vi "Begin.vi"() -> (0 "error out":errorcluster, 1 "CameraDevRef":T1)   [LabVIEW 2011]
doc: "Called before other user functions, this VI is expected to open initial I/O refnums, load in file data, and do all program initialization. Notice that the <B>error out</B> terminal is simply used for data flow. Wiring it to other structures or subVIs ensures that this VI runs first."
uses:
  <vilib>/Rock Robotics/WPI/Camera/WPI_CameraDevRef.ctl
  <vilib>/Rock Robotics/SystemInterfaces/DIO/FPGA_DIOPWMChannel.ctl
  <vilib>/Rock Robotics/WPI/Joystick/WPI_JoystickDeviceEnum.ctl
  <vilib>/Rock Robotics/WPI/Relay/WPI_RelayDirection.ctl
  <vilib>/Rock Robotics/SystemInterfaces/DIO/FPGA_DIORelayChannel.ctl
  <vilib>/Rock Robotics/SystemInterfaces/Typedef/FPGA_TypedefDigitalModule.ctl
  <vilib>/Rock Robotics/SystemInterfaces/AI/FPGA_AIChannel.ctl
  <vilib>/Rock Robotics/SystemInterfaces/DIO/FPGA_DIOChannel.ctl
  <vilib>/Rock Robotics/WPI/Encoder/WPI_EncoderType.ctl
  <vilib>/Rock Robotics/SystemInterfaces/AI/FPGA_AIGyroChannel.ctl
  <vilib>/Rock Robotics/WPI/MotorControl/WPI_MotorControlOpen Jaguar.vi
  <vilib>/Rock Robotics/WPI/MotorControl/WPI_MotorControlOpen Victor.vi
  Robot Global Data.vi
  <vilib>/Rock Robotics/WPI/Counter/WPI_CounterDigitalInputToDigitalSource.vi
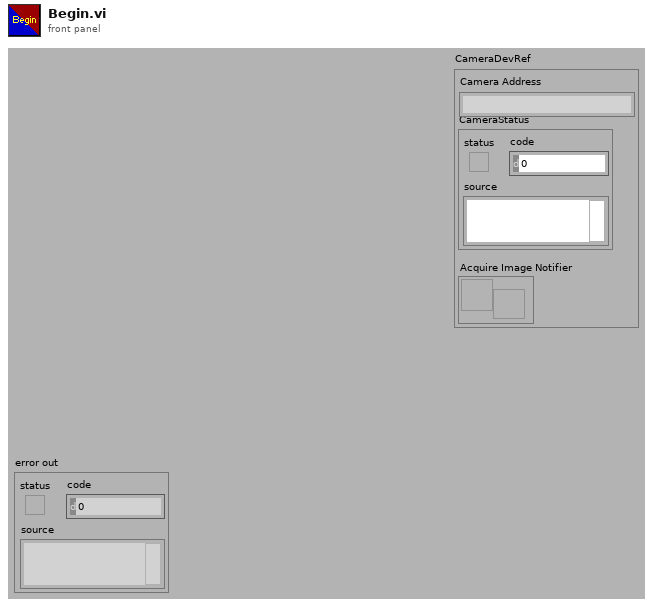
[diagram p1: front panel]
types:
  T1 = typedef "WPI_CameraDevRef.ctl" = cluster{"Camera Address":string, "CameraStatus":errorcluster, "Acquire Image Notifier":refnum<notifier>}
  T2 = typedef "FPGA_AIGyroChannel.ctl" = enum8{"AI 1", "AI 2", "Invalid"}
  T3 = typedef "WPI_EncoderType.ctl" = enum16{"1x", "2x", "4x"}
  T4 = typedef "FPGA_DIOChannel.ctl" = enum8{"DIO 1", "DIO 2", "DIO 3", "DIO 4", "DIO 5", "DIO 6", "DIO 7", "DIO 8", "DIO 9", "DIO 10", "DIO 11", "DIO 12", "DIO 13", "DIO 14", "Invalid"}
  T5 = typedef "FPGA_AIChannel.ctl" = enum8{"AI 1", "AI 2", "AI 3", "AI 4", "AI 5", "AI 6", "AI 7", "AI 8", "Invalid"}
  T6 = typedef "FPGA_TypedefDigitalModule.ctl" = enum16{"Digital Module 1", "Digital Module 2"}
  T7 = typedef "FPGA_DIORelayChannel.ctl" = enum8{"Relay 1", "Relay 2", "Relay 3", "Relay 4", "Relay 5", "Relay 6", "Relay 7", "Relay 8", "Invalid"}
  T8 = typedef "WPI_RelayDirection.ctl" = enum16{"Both directions", "Forward only", "Reverse only"}
  T9 = typedef "WPI_JoystickDeviceEnum.ctl" = enum16{"USB 1", "USB 2", "USB 3", "USB 4", "Kinect 1", "Kinect 2"}
  T10 = typedef "FPGA_DIOPWMChannel.ctl" = enum8{"PWM 1", "PWM 2", "PWM 3", "PWM 4", "PWM 5", "PWM 6", "PWM 7", "PWM 8", "PWM 9", "PWM 10", "Invalid"}
  T11 = typedef "WPI_CameraImageSize.ctl" = enum16{"640x480", "320x240", "160x120"}
  T12 = cluster{"fps":i32, "compression":i32, "Image Size":T11}
  T13 = typedef "WPI_I2CDevRef.ctl" = cluster{"DevStatus":errorcluster, "Digital Module":T6, "Device Address":u8}
  T14 = typedef "WPI_DigitalInputDevRef.ctl" = cluster{"DevStatus":errorcluster, "DIO Channel":T4, "Digital Module":T6}
  T15 = typedef "FPGA_CounterEncoderSourceConvertionLVSourceType.ctl" = cluster{"DevStatus":errorcluster, "AnalogTriggerMode?":bool, "DigitalMode":cluster{"Digital Module":T6, "DIO Channel":T16}, "AnalogTriggerMode":cluster{"AnalogTriggerIndex":T17, "OutputType":T18}}
  T16 = typedef "FPGA_DIODigitalSourceChannel.ctl" = enum8{"DIO 1", "DIO 2", "DIO 3", "DIO 4", "DIO 5", "DIO 6", "DIO 7", "DIO 8", "DIO 9", "DIO 10", "DIO 11", "DIO 12", "DIO 13", "DIO 14", "Disabled"}
  T17 = typedef "FPGA_AnalogTriggerIndex.ctl" = enum8{"Trig 0", "Trig 1", "Trig 2", "Trig 3", "Trig 4", "Trig 5", "Trig 6", "Trig 7", "Invalid"}
  T18 = typedef "FPGA_AnalogTriggerOutType.ctl" = enum16{"InWindow", "TriggerState", "Rising", "Falling"}
  T19 = typedef "WPI_EncoderDevRef.ctl" = cluster{"DevStatus":errorcluster, "EncoderIndex":T20, "CounterIndex":T21, "DistancePerCount":dbl, "Decoding Type":T3}
  T20 = typedef "FPGA_EncoderIdx.ctl" = enum8{"Enc 0", "Enc 1", "Enc 2", "Enc 3", "Invalid"}
  T21 = typedef "FPGA_CounterCtrSystemIndex.ctl" = enum8{"Ctr 0", "Ctr 1", "Ctr 2", "Ctr 3", "Ctr 4", "Ctr 5", "Ctr 6", "Ctr 7", "Invalid"}
  T22 = typedef "WPI_CameraWhite Balance Values.ctl" = enum16{"Auto", "Fixed indoor", "Fixed outdoor 1", "Fixed outdoor 2", "Fixed fluorescent 1", "Fixed fluorescent 2", "Hold current"}
  T23 = typedef "WPI_CameraExposure Values.ctl" = enum16{"Auto", "Flicker-free 50 Hz", "Flicker-free 60 Hz", "Hold current"}
  T24 = typedef "WPI_ServoDeviceRef.ctl" = cluster{"DeviceStatus":errorcluster, "Digital Module":T6, "PWM Channel":T10, "DeadBand":T25}
  T25 = typedef "WPI_PWMDeadband.ctl" = cluster{"Name":string, "maxPositivePwm":i32, "minPositivePwm":i32, "centerPwm":i32, "maxNegativePwm":i32, "minNegativePwm":i32, "angularRange":u16}
  T26 = typedef "WPI_MotorControlDeviceRef.ctl" = cluster{"DeviceStatus":errorcluster, "Type":enum16{"PWM", "CAN"}, "PWM":cluster{"Digital Module":T6, "PWM Channel":T10, "DeadBand":T25}, "CAN":cluster{"Device Number":u8, "Control Mode":T27, "Semaphore":T28, "Max Vout":dbl}, "Invert":bool, "TransformRef":T29, "InvTransformRef":T29}
  T27 = typedef "WPI_CANJaguar_ControlMode.ctl" = enum8{"Percent VBus", "Current", "Speed", "Position", "Voltage"}
  T28 = typedef "Semaphore RefNum" = refnum<k1>
  T29 = typedef "WPI_PWMTransform_ConPane.ctl" = refnum<vi>
  T30 = typedef "WPI_AnalogChannelDevRef.ctl" = cluster{"DevStatus":errorcluster, "Analog Module":T31, "Analog Channel":T5}
  T31 = typedef "FPGA_TypedefAnalogModule.ctl" = enum16{"Analog Module 1", "Analog Module 2"}
  T32 = typedef "WPI_JoystickDevRef.ctl" = cluster{"Device":T9}
  T33 = typedef "WPI_GyroDevRef.ctl" = cluster{"DevStatus":errorcluster, "Analog Module":T31, "Analog Channel":T5, "Offset":dbl, "Gain (VoltsPerDegree/Second)":dbl}
  T34 = typedef "WPI_RelayDevRef.ctl" = cluster{"DevStatus":errorcluster, "Relay Channel":T7, "Digital Module":T6, "Relay Direction":T8}
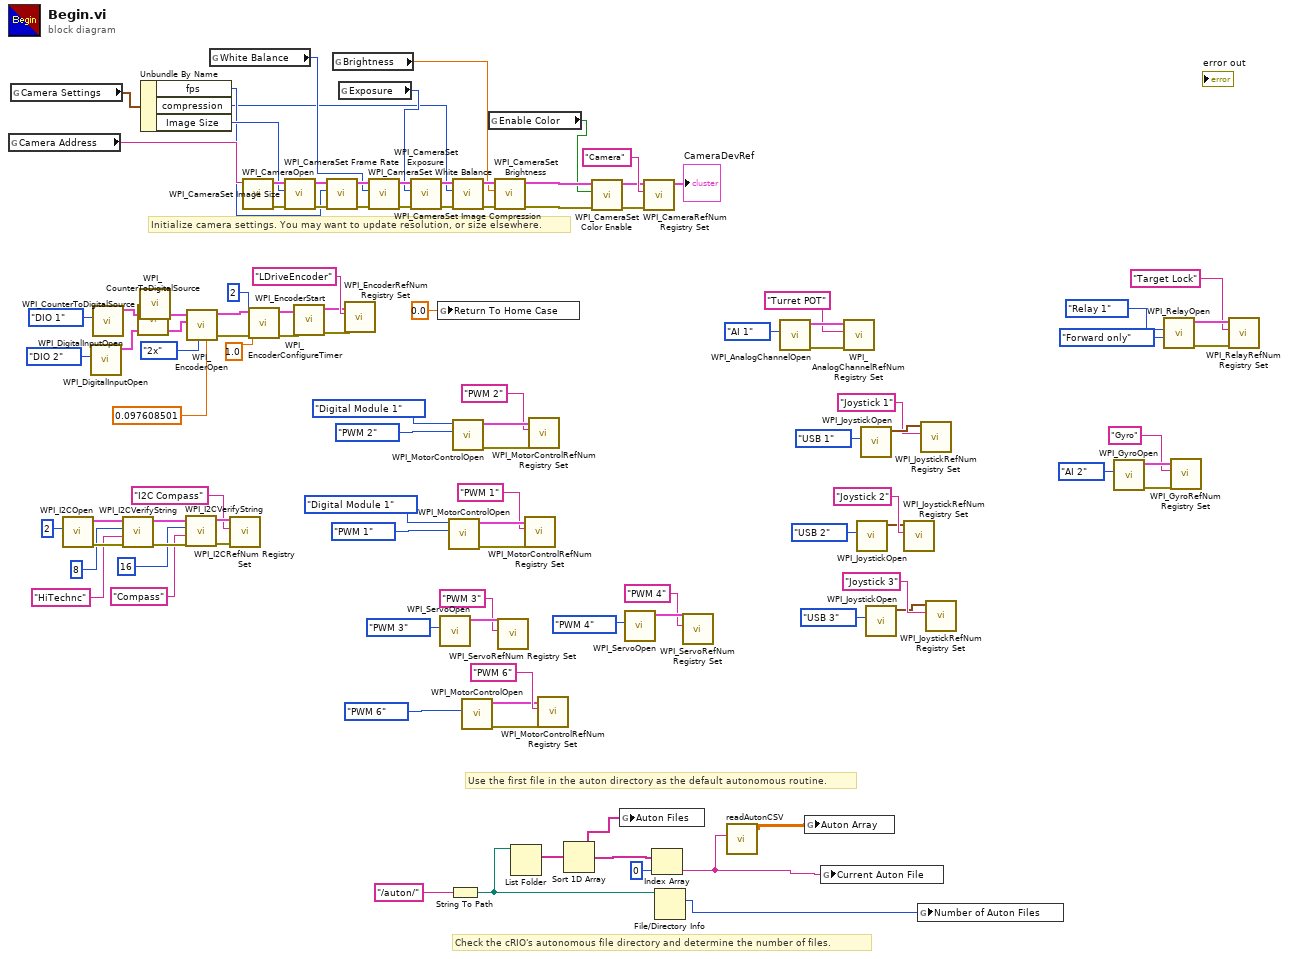
[diagram p0: block diagram]
diagram:
  # "Check the cRIO's autonomous file directory and determine the number of files."
  # "Use the first file in the auton directory as the default autonomous routine."
  # "Initialize camera settings. You may want to update resolution, or size elsewhere."
  n1 = global read "Robot Global Data.vi" "Camera Address"() -> (w94:string)
  n2 = global read "Robot Global Data.vi" "Camera Settings"() -> (w66:T12)
  n3 = call <vilib>:"WPI_I2COpen.vi"("Device Address"=u8 2) -> ("error out"=w12:errorcluster, "I2CDevRef"=w11:T13)  [unwired: 9 in]
  n4 = call <vilib>:"WPI_DigitalInputOpen.vi"("DIO Channel"=FPGA_DIOChannel."DIO 2") -> ("DigitalInputDevRef"=w29:T14)  [unwired: 9 in, 1 out]
  n5 = call <vilib>:"WPI_DigitalInputOpen.vi"("DIO Channel"=FPGA_DIOChannel."DIO 1") -> ("DigitalInputDevRef"=w32:T14)  [unwired: 9 in, 1 out]
  n6 = call <vilib>:"WPI_I2CVerifyString.vi"("error in (no error)"=w12, "Expected"="HiTechnc", "Register Address"=u8 8, "I2CDevRef"=w11) -> ("error out"=w10:errorcluster, "I2CDevRef"=w9:T13)  [unwired: 6 in]
  n7 = call-poly <vilib>:"WPI_CounterToDigitalSource.vi"("DigitalInputDevRef"=w29) -> ("Digital Source"=w28:T15)  [unwired: 6 in]
  n8 = call-poly <vilib>:"WPI_CounterToDigitalSource.vi"("DigitalInputDevRef"=w32) -> ("Digital Source"=w33:T15)  [unwired: 6 in]
  n9 = Unbundle By Name(w66) -> ("fps"=w64:i32, "compression"=w61:i32, "Image Size"=w65:T11)
  n10 = call <vilib>:"WPI_I2CVerifyString.vi"("error in (no error)"=w10, "Expected"="Compass", "Register Address"=u8 16, "I2CDevRef"=w9) -> ("error out"=w8:errorcluster, "I2CDevRef"=w7:T13)  [unwired: 6 in]
  n11 = call <vilib>:"WPI_EncoderOpen.vi"("DistancePerCount"=0.097608501, "Decoding Type"=WPI_EncoderType."2x", "BSource"=w28, "ASource"=w33) -> ("error out"=w24:errorcluster, "EncoderDevRef"=w23:T19)  [unwired: 6 in]
  n12 = global read "Robot Global Data.vi" "White Balance"() -> (w63:T22)
  n13 = call <vilib>:"WPI_I2CRefNum Registry Set.vi"("error in (no error)"=w8, "refnum name"="I2C Compass", "I2CDevRef"=w7) -> ()  [unwired: 7 in, 2 out]
  n14 = call <vilib>:"WPI_CameraOpen.vi"("Camera Address"=w94) -> ("error out"=w100:errorcluster, "CameraDevRef"=w101:T1)  [unwired: 1 in, 8 out]
  n15 = call <vilib>:"WPI_EncoderConfigureTimer.vi"("error in (no error)"=w24, "Number Samples to Average"=u8 2, "Minimum Rate"=1.0, "EncoderDevRef"=w23) -> ("error out"=w19:errorcluster, "EncoderDevRef"=w20:T19)  [unwired: 6 in]
  n16 = call <vilib>:"WPI_CameraSet Image Size.vi"("error in (no error)"=w100, "Image Size"=w65, "CameraDevRef"=w101) -> ("error out"=w99:errorcluster, "CameraDevRef Out"=w102:T1)  [unwired: 7 out]
  n17 = call <vilib>:"WPI_EncoderStart.vi"("error in (no error)"=w19, "EncoderDevRef"=w20) -> ("error out"=w17:errorcluster, "EncoderDevRef"=w18:T19)  [unwired: 8 in]
  n18 = call <vilib>:"WPI_CameraSet Frame Rate.vi"("error in (no error)"=w99, "Frame Rate (fps)"=w64, "CameraDevRef"=w102) -> ("error out"=w98:errorcluster, "CameraDevRef Out"=w104:T1)  [unwired: 7 out]
  n19 = global read "Robot Global Data.vi" "Brightness"() -> (w60:dbl)
  n20 = global read "Robot Global Data.vi" "Exposure"() -> (w62:T23)
  n21 = call <vilib>:"WPI_EncoderRefNum Registry Set.vi"("error in (no error)"=w17, "refnum name"="LDriveEncoder", "EncoderDevRef"=w18) -> ()  [unwired: 7 in, 2 out]
  n22 = call <vilib>:"WPI_CameraSet White Balance.vi"("error in (no error)"=w98, "White Balance"=w63, "CameraDevRef"=w104) -> ("error out"=w97:errorcluster, "CameraDevRef Out"=w103:T1)  [unwired: 7 out]
  n23 = call <vilib>:"WPI_CameraSet Exposure.vi"("error in (no error)"=w97, "Exposure"=w62, "CameraDevRef"=w103) -> ("error out"=w96:errorcluster, "CameraDevRef Out"=w106:T1)  [unwired: 7 out]
  n24 = global write "Robot Global Data.vi" "Return To Home Case"(0.0 ("Return To Home Case")) -> ()
  n25 = call <vilib>:"WPI_ServoOpen.vi"("PWM Channel"=FPGA_DIOPWMChannel."PWM 3") -> ("ServoDeviceRef"=w80:T24)  [unwired: 9 in, 1 out]
  n26 = call-poly <vilib>:"WPI_MotorControlOpen.vi"("PWM Channel"=FPGA_DIOPWMChannel."PWM 1", "Digital Module (Module 1)"=FPGA_TypedefDigitalModule."Digital Module 1") -> ("error out"=w86:errorcluster, "MotorControlDeviceRef"=w89:T26)  [unwired: 8 in]
  n27 = String To Path(string="/auton/") -> (path=w40:path)
  n28 = call <vilib>:"WPI_CameraSet Image Compression.vi"("error in (no error)"=w96, "Compression"=w61, "CameraDevRef"=w106) -> ("error out"=w95:errorcluster, "CameraDevRef Out"=w105:T1)  [unwired: 7 out]
  n29 = call-poly <vilib>:"WPI_MotorControlOpen.vi"("PWM Channel"=FPGA_DIOPWMChannel."PWM 2", "Digital Module (Module 1)"=FPGA_TypedefDigitalModule."Digital Module 1") -> ("error out"=w87:errorcluster, "MotorControlDeviceRef"=w92:T26)  [unwired: 8 in]
  n30 = call-poly <vilib>:"WPI_MotorControlOpen.vi"("PWM Channel"=FPGA_DIOPWMChannel."PWM 6") -> ("error out"=w75:errorcluster, "MotorControlDeviceRef"=w73:T26)  [unwired: 9 in]
  n31 = global read "Robot Global Data.vi" "Enable Color"() -> (w55:bool)
  n32 = call <vilib>:"WPI_CameraSet Brightness.vi"("error in (no error)"=w95, "Brightness"=w60, "CameraDevRef"=w105) -> ("error out"=w58:errorcluster, "CameraDevRef Out"=w59:T1)  [unwired: 7 out]
  n33 = call <vilib>:"WPI_ServoRefNum Registry Set.vi"("refnum name"="PWM 3", "ServoDeviceRef"=w80) -> ()  [unwired: 8 in, 2 out]
  n34 = List Folder(path=w40) -> (filenames=w39:string[])  [unwired: 1 in, 5 out]
  n35 = call <vilib>:"WPI_MotorControlRefNum Registry Set.vi"("error in (no error)"=w86, "refnum name"="PWM 1", "MotorControlDevRef"=w89) -> ()  [unwired: 7 in, 2 out]
  n36 = call <vilib>:"WPI_MotorControlRefNum Registry Set.vi"("error in (no error)"=w87, "refnum name"="PWM 2", "MotorControlDevRef"=w92) -> ()  [unwired: 7 in, 2 out]
  n37 = call <vilib>:"WPI_MotorControlRefNum Registry Set.vi"("error in (no error)"=w75, "refnum name"="PWM 6", "MotorControlDevRef"=w73) -> ()  [unwired: 7 in, 2 out]
  n38 = Sort 1D Array(array=w39) -> (sorted array=w34:string[])
  n39 = call <vilib>:"WPI_CameraSet Color Enable.vi"("error in (no error)"=w58, "Color Enabled"=w55, "CameraDevRef"=w59) -> ("error out"=w56:errorcluster, "CameraDevRef Out"=w57:T1)  [unwired: 7 in]
  n40 = global write "Robot Global Data.vi" "Auton Files"(w34) -> ()
  n41 = call <vilib>:"WPI_ServoOpen.vi"("PWM Channel"=FPGA_DIOPWMChannel."PWM 4") -> ("ServoDeviceRef"=w78:T24)  [unwired: 9 in, 1 out]
  n42 = call <vilib>:"WPI_CameraRefNum Registry Set.vi"("error in (no error)"=w56, "refnum name"="Camera", "CameraDevRef"=w57) -> ("CameraDevRef"=→"CameraDevRef":T1)  [unwired: 8 out]
  n43 = Index Array(array=w34, index=0) -> (element=w36:string)
  n44 = File/Directory Info(path=w40) -> (size=w37:i64)  [unwired: 1 in, 6 out]
  n45 = call <vilib>:"WPI_ServoRefNum Registry Set.vi"("refnum name"="PWM 4", "ServoDeviceRef"=w78) -> ()  [unwired: 8 in, 2 out]
  n46 = call "readAutonCSV.vi"("AutonFile"=w36) -> ("AutonArray"=w35:dbl[][])  [unwired: 7 in]
  n47 = call <vilib>:"WPI_AnalogChannelOpen.vi"("Analog Channel"=FPGA_AIChannel."AI 1") -> ("error out"=w45:errorcluster, "AIDeviceRef"=w46:T30)  [unwired: 9 in]
  n48 = global write "Robot Global Data.vi" "Auton Array"(w35) -> ()
  n49 = global write "Robot Global Data.vi" "Current Auton File"(w36) -> ()
  n50 = call <vilib>:"WPI_AnalogChannelRefNum Registry Set.vi"("error in (no error)"=w45, "refnum name"="Turret POT", "AIDeviceRef"=w46) -> ()  [unwired: 7 in, 2 out]
  n51 = call <vilib>:"WPI_JoystickOpen.vi"("JoystickDevice"=WPI_JoystickDeviceEnum."USB 2") -> ("JoystickDevRef"=w82:T32)  [unwired: 10 in]
  n52 = call <vilib>:"WPI_JoystickOpen.vi"("JoystickDevice"=WPI_JoystickDeviceEnum."USB 1") -> ("JoystickDevRef"=w85:T32)  [unwired: 10 in]
  n53 = call <vilib>:"WPI_JoystickOpen.vi"("JoystickDevice"=WPI_JoystickDeviceEnum."USB 3") -> ("JoystickDevRef"=w70:T32)  [unwired: 10 in]
  n54 = call <vilib>:"WPI_JoystickRefNum Registry Set.vi"("refnum name"="Joystick 2", "JoystickDevRef"=w82) -> ()  [unwired: 8 in, 2 out]
  n55 = global write "Robot Global Data.vi" "Number of Auton Files"(w37) -> ()
  n56 = call <vilib>:"WPI_JoystickRefNum Registry Set.vi"("refnum name"="Joystick 1", "JoystickDevRef"=w85) -> ()  [unwired: 8 in, 2 out]
  n57 = call <vilib>:"WPI_JoystickRefNum Registry Set.vi"("refnum name"="Joystick 3", "JoystickDevRef"=w70) -> ()  [unwired: 8 in, 2 out]
  n58 = call <vilib>:"WPI_GyroOpen.vi"("Analog Channel"=FPGA_AIGyroChannel."AI 2") -> ("error out"=w16:errorcluster, "GyroDevRef"=w15:T33)  [unwired: 8 in, 1 out]
  n59 = call <vilib>:"WPI_RelayOpen.vi"("Relay Direction"=WPI_RelayDirection."Forward only", "Relay Channel"=FPGA_DIORelayChannel."Relay 1") -> ("error out"=w52:errorcluster, "RelayDevRef"=w53:T34)  [unwired: 8 in]
  n60 = call <vilib>:"WPI_GyroRefNum Registry Set.vi"("error in (no error)"=w16, "refnum name"="Gyro", "GyroDevRef"=w15) -> ()  [unwired: 7 in, 2 out]
  n61 = call <vilib>:"WPI_RelayRefNum Registry Set.vi"("error in (no error)"=w52, "refnum name"="Target Lock", "RelayDevRef"=w53) -> ()  [unwired: 7 in, 2 out]
